vi "SplitHTTPHeaders.vi"(4 "error in (no error)":errorcluster, 7 "HTTP Header String":string) -> (0 "error out":errorcluster, 2 "Header Array":cluster{"Name":string, "Value":string}[](array[cluster]), 3 "HTTP Request":string)   [LabVIEW 2015, in "WebSockets.lvlib"]
doc: "Returns the remaining HTTP headers received from the client.\nWebSockets API 1.3.0.13\nSam Sharp - Intelligent Energy\nCopyright (c) 2015, Intelligent Energy"
uses:
  WebSockets.lvlib
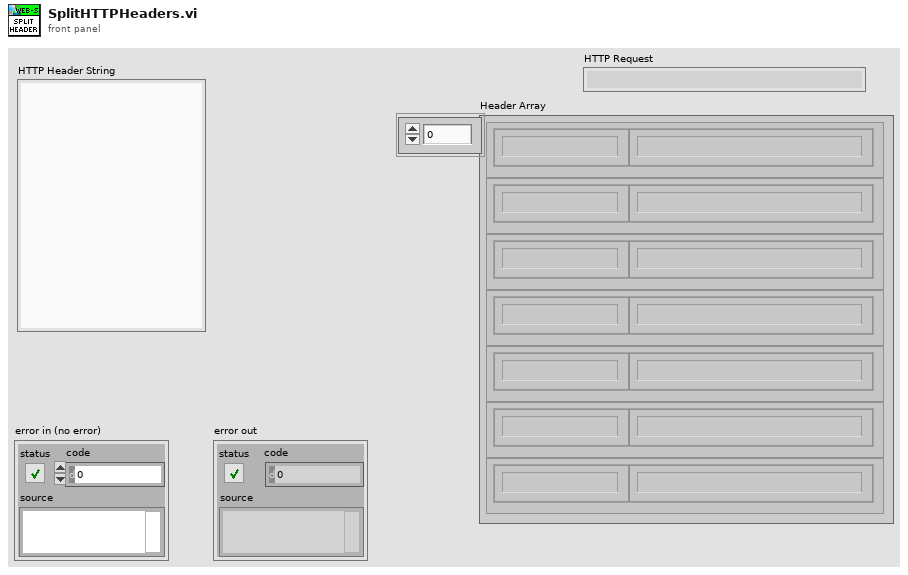
[diagram p1: front panel]
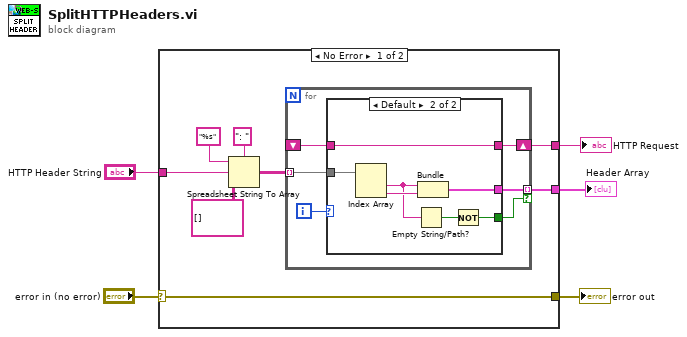
[diagram p0: block diagram]
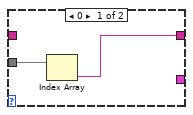
[diagram p2: hidden frame]
diagram:
  n1 = case shown="No Error" "error in (no error)" {
    selector: "error in (no error)" -> [w9 w29]
    tunnel: "HTTP Header String" -> [w11 _]
    tunnel: [w9 w29] -> w3
    tunnel: [w7 _] -> w2
    tunnel: [w6 _] -> w1
    frame No Error {
      n2 = Spreadsheet String To Array(delimiter (Tab)=": ", format string="%s", spreadsheet string=w11, array type (2D Dbl)=string[][] []) -> (array=w8:string[][])
      n3 = for {
        tunnel: w8 -> [w18] mode=indexing
        tunnel: [w17] -> w7 mode=indexing if=w16
        shift-right: [w15] -> w6
        shift-left: _ -> [w14]
        i -> [w19]
        n4 = case shown="Default" w19 {
          tunnel: w18 -> [w21 w28]
          tunnel: [_ w26] -> w17
          tunnel: [_ w22] -> w16
          tunnel: [w20 w25] -> w15
          tunnel: w14 -> [_ w25]
          frame 0 {
            n5 = Index Array(array=w21) -> (element=w20:string)  [unwired: 1 in]
          }
          frame Default {
            n6 = Index Array(array=w28) -> (element #1=w24:string, element #2=w27:string)  [unwired: 2 in]
            n7 = Empty String/Path?(string/path=w24) -> (empty?=w23:bool)
            n8 = Bundle(w24, w27) -> (w26:cluster{string, string})  [unwired: 1 in]
            n9 = Not(x=w23) -> (.not. x?=w22:bool)
          }
        }
      }
    }
    frame Error {
    }
  }
  "HTTP Request" <- w1
  "error out" <- w3
  "Header Array" <- w2
